vi "DriverStationPushData.vi"   [LabVIEW 2018]
uses:
  dsdata.vi
  constants.vi
  <vilib>/Rock Robotics/Network Tables/NT Write String Array.vi
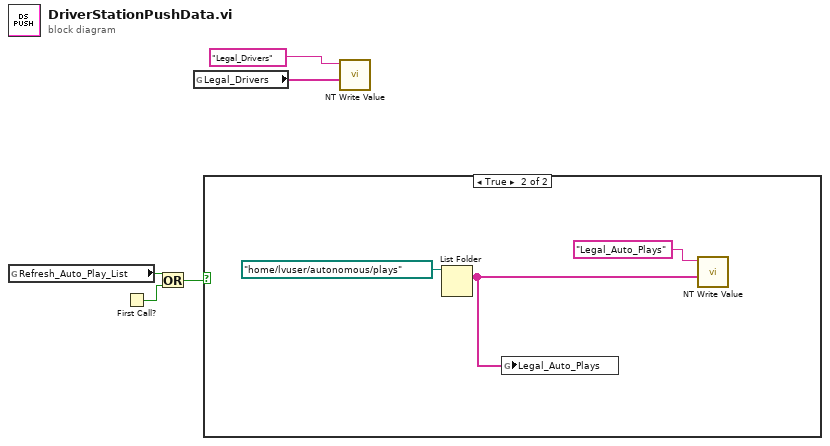
[diagram p0: block diagram]
diagram:
  n1 = global read "dsdata.vi" "Refresh_Auto_Play_List"() -> (w3:bool)
  n2 = First Call?() -> (First Call?: T/F=w2:bool)
  n3 = Or(x=w3, y=w2) -> (x .or. y?=w1:bool)
  n4 = global read "constants.vi" "Legal_Drivers"() -> (w5:string[])
  n5 = case shown="True" w1 {
    frame False {
    }
    frame True {
      n6 = List Folder(path=path "/home/lvuser/autonomous/plays") -> (filenames=w6:string[])  [unwired: 3 in, 3 out]
      n7 = global write "constants.vi" "Legal_Auto_Plays"(w6) -> ()
      n8 = call-poly <vilib>:"NT Write Value.vi"("String Array"=w6, "Name"="Legal_Auto_Plays") -> ()  [unwired: 9 in, 1 out]
    }
  }
  n9 = call-poly <vilib>:"NT Write Value.vi"("String Array"=w5, "Name"="Legal_Drivers") -> ()  [unwired: 9 in, 1 out]
